vi "HFRR ADV v036 new software.vi"() -> ()   [LabVIEW 2025] (continued)
                        n2404 = local write "EVENT LOG"(w3467) -> ()
                      }
                      frame #22 {
                        n2405 = Wait (ms)(milliseconds to wait=u32 50) -> ()  [unwired: 1 out]
                      }
                      frame #23 {
                        n2406 = local read "NORMAL LOAD"() -> (w3471:dbl)
                        n2407 = Number To Fractional String(number=w3471, precision (6)=i16 2) -> (F-format string=w3472:string)  [unwired: 2 in]
                        n2408 = Concatenate Strings("Applied Load [grams] :" ("Content"), w3472) -> (w3474:string)
                        n2409 = local read "EVENT LOG"() -> (w3476:string)
                        n2410 = call "Event Log.vi"("Content"=w3474, "EVENT LOG"=w3476) -> ("EVENT LOG"=w3475:string)  [unwired: 8 in, 1 out]
                        n2411 = local write "EVENT LOG"(w3475) -> ()
                      }
                      frame #24 {
                        n2412 = Wait (ms)(milliseconds to wait=u32 50) -> ()  [unwired: 1 out]
                      }
                      frame #25 {
                        n2413 = local read "Set Strk"() -> (w3479:dbl)
                        n2414 = Number To Fractional String(number=w3479, precision (6)=i16 2) -> (F-format string=w3480:string)  [unwired: 2 in]
                        n2415 = Concatenate Strings("Set Stroke [mm] :" ("Content"), w3480) -> (w3482:string)
                        n2416 = local read "EVENT LOG"() -> (w3484:string)
                        n2417 = call "Event Log.vi"("Content"=w3482, "EVENT LOG"=w3484) -> ("EVENT LOG"=w3483:string)  [unwired: 8 in, 1 out]
                        n2418 = local write "EVENT LOG"(w3483) -> ()
                      }
                      frame #26 {
                        n2419 = Wait (ms)(milliseconds to wait=u32 50) -> ()  [unwired: 1 out]
                      }
                      frame #27 {
                        n2420 = local read "Set Temp"() -> (w3487:dbl)
                        n2421 = Number To Fractional String(number=w3487, precision (6)=i16 2) -> (F-format string=w3488:string)  [unwired: 2 in]
                        n2422 = Concatenate Strings("Set Temperature [deg C] :" ("Content"), w3488) -> (w3490:string)
                        n2423 = local read "EVENT LOG"() -> (w3492:string)
                        n2424 = call "Event Log.vi"("Content"=w3490, "EVENT LOG"=w3492) -> ("EVENT LOG"=w3491:string)  [unwired: 8 in, 1 out]
                        n2425 = local write "EVENT LOG"(w3491) -> ()
                      }
                      frame #28 {
                        n2426 = Wait (ms)(milliseconds to wait=u32 50) -> ()  [unwired: 1 out]
                      }
                      frame #29 {
                        n2427 = local read "Set Rh"() -> (w3495:dbl)
                        n2428 = Number To Fractional String(number=w3495, precision (6)=i16 2) -> (F-format string=w3496:string)  [unwired: 2 in]
                        n2429 = Concatenate Strings("Set Humidity [%RH] :" ("Content"), w3496) -> (w3498:string)
                        n2430 = local read "EVENT LOG"() -> (w3500:string)
                        n2431 = call "Event Log.vi"("Content"=w3498, "EVENT LOG"=w3500) -> ("EVENT LOG"=w3499:string)  [unwired: 8 in, 1 out]
                        n2432 = local write "EVENT LOG"(w3499) -> ()
                      }
                      frame #30 {
                        n2433 = Wait (ms)(milliseconds to wait=u32 50) -> ()  [unwired: 1 out]
                      }
                      frame #31 {
                        n2434 = local read "test time"() -> (w3503:dbl)
                        n2435 = Number To Fractional String(number=w3503, precision (6)=i16 1) -> (F-format string=w3504:string)  [unwired: 2 in]
                        n2436 = Concatenate Strings("Test Duration [mins] :" ("Content"), w3504) -> (w3506:string)
                        n2437 = local read "EVENT LOG"() -> (w3508:string)
                        n2438 = call "Event Log.vi"("Content"=w3506, "EVENT LOG"=w3508) -> ("EVENT LOG"=w3507:string)  [unwired: 8 in, 1 out]
                        n2439 = local write "EVENT LOG"(w3507) -> ()
                      }
                      frame #32 {
                        w3509 = dbl[] [] ("History Data")
                        w3510 = cluster{"y":dbl, dbl, "y":dbl}[] [] ("History Data")
                        w3511 = FALSE ("Visible")
                        n2440 = property on="Stroke ( mm )" class="WFChart (strict)"("History Data"=w3510) -> ()  [unwired: 2 in, 2 out]
                        n2441 = property on="Humidity ( %RH ) 2" class="WFChart (strict)"("History Data"=w3509) -> ()  [unwired: 2 in, 2 out]
                        n2442 = property on="Temperature ( Deg C )" class="WFChart (strict)"("History Data"=w3509) -> ()  [unwired: 2 in, 2 out]
                        n2443 = property on="Electrical Contact Resistance ( % )" class="WFChart (strict)"("History Data"=w3509) -> ()  [unwired: 2 in, 2 out]
                        n2444 = property on="Coefficient of Friction" class="WFChart (strict)"("History Data"=w3509) -> ()  [unwired: 2 in, 2 out]
                        n2445 = property on="Frictional Force ( N )" class="WFChart (strict)"("History Data"=w3509) -> ()  [unwired: 2 in, 2 out]
                        n2446 = property on="Coefficient of Friction" class="WFChart (strict)"("History Data"=w3509) -> ()  [unwired: 2 in, 2 out]
                        n2447 = property on="Frictional Force ( N )" class="WFChart (strict)"("History Data"=w3509) -> ()  [unwired: 2 in, 2 out]
                        n2448 = property on="Electrical Contact Resistance ( % )" class="WFChart (strict)"("History Data"=w3509) -> ()  [unwired: 2 in, 2 out]
                        n2449 = property on="Stroke ( mm )" class="WFChart (strict)"("History Data"=w3510) -> ()  [unwired: 2 in, 2 out]
                        n2450 = property on="Temperature ( Deg C )" class="WFChart (strict)"("History Data"=w3509) -> ()  [unwired: 2 in, 2 out]
                        n2451 = property on="Service Password Log" class="Str"("Visible"=w3511) -> ()  [unwired: 2 in, 2 out]
                        n2452 = property on="Password 3" class="Clust (strict)"("Visible"=w3511) -> ()  [unwired: 2 in, 2 out]
                      }
                    }
                    "TEST FILE NAM,E SAVED" <- TRUE ("TEST FILE NAM,E SAVED")
                  }
                }
              }
            }
          }
        }
        n2453 = local write "Test \nStatus"(w2890) -> ()
        n2454 = local write "Save"(w2890) -> ()
        n2455 = local read "Main Tab"() -> (w2884:T2)
        n2456 = case shown="True" w2887 {
          frame False {
            n2457 = local read "Rt 3"() -> (w2955:bool)
            n2458 = case shown="True" w2955 {
              frame False {
              }
              frame True {
                n2459 = local write "Rt 3"(FALSE ("Rt 3")) -> ()
              }
            }
            "Rt" <- TRUE ("Rt")
            "Rt 2" <- FALSE ("Rt")
          }
          frame True {
            n2460 = local read "Rt"() -> (w2961:bool)
            n2461 = local write "Rt 2"(TRUE ("Rt 2")) -> ()
            n2462 = case shown="True" w2961 {
              frame False {
              }
              frame True {
                n2463 = local write "Rt"(FALSE ("Rt")) -> ()
              }
            }
            "Rt 3" <- TRUE ("Rt 3")
          }
        }
        n2464 = case shown="\"Acquire\"" w2884 {
          tunnel: w2886 -> [_ w2990]
          frame Default {
            w2989 = 0.0 ("output")
            n2465 = local write "PID-out"(w2989) -> ()
            n2466 = local write "Frequency ( Hz )"(w2989) -> ()
            n2467 = local write "STROKE Initialize"(TRUE ("STROKE Initialize")) -> ()
          }
          frame "Acquire" {
            n2468 = stacked-sequence {
              frame #0 {
                n2469 = local read "Auto Start Test"() -> (w2992:bool)
                n2470 = case shown="True" w2992 {
                  tunnel: "RUN" -> [w3013 w3016]
                  tunnel: [w3013 w3015] -> w2993
                  frame False {
                  }
                  frame True {
                    n2471 = local read "Auto Start Temp"() -> (w3014:bool)
                    n2472 = Or(x=w3016, y=w3014) -> (x .or. y?=w3015:bool)
                  }
                }
                n2473 = local read "clk"() -> (w3012:dbl)
                n2474 = local read "Save"() -> (w3008:bool)
                n2475 = Equal?(x=w3012, y=0.0) -> (x = y?=w3009:bool)
                n2476 = And(x=w3009, y=w3008) -> (x .and. y?=w3010:bool)
                n2477 = Not(x="Engage") -> (.not. x?=w2999:bool)
                n2478 = case shown="False" w2993 {
                  tunnel: [0.0 w3039] -> w2995
                  frame False {
                    (unwired) TRUE ("Visible")
                    n2479 = local read "Auto Start Test"() -> (w3020:bool)
                    n2480 = local write "Start Time"(TRUE ("Start Time")) -> ()
                    n2481 = property on="Stroke 2" class="DigNum (strict)"("Visible"=FALSE) -> ()  [unwired: 2 in, 2 out]
                    n2482 = case shown="False" w3020 {
                      frame False {
                        n2483 = property on="Heater Button" class="Bool (strict)"("DisabledEnum"=T19."Enabled" ("Disabled")) -> ()  [unwired: 2 in, 2 out]
                        n2484 = property on="Humidity" class="Bool (strict)"("DisabledEnum"=T19."Enabled" ("Disabled")) -> ()  [unwired: 2 in, 2 out]
                      }
                      frame True {
                      }
                    }
                    n2485 = case shown="False" "TestCompFlg" {
                      frame False {
                        n2486 = local read "StartFlg"() -> (w3028:bool)
                        n2487 = case shown="True" w3028 {
                          frame False {
                          }
                          frame True {
                            n2488 = stacked-sequence {
                              frame #0 {
                                n2489 = local read "EVENT LOG"() -> (w3032:string)
                                n2490 = call "Event Log.vi"("Content"="Test was interrupted", "EVENT LOG"=w3032) -> ("EVENT LOG"=w3033:string)  [unwired: 8 in, 1 out]
                                n2491 = local write "EVENT LOG"(w3033) -> ()
                                n2492 = property on="RUN" class="Bool (strict)"("Visible"=TRUE) -> ()  [unwired: 2 in, 2 out]
                                n2493 = property on="Auto Start Test" class="Bool (strict)"("Visible"=TRUE) -> ()  [unwired: 2 in, 2 out]
                              }
                              frame #1 {
                                w3035 = FALSE ("StartFlg")
                                n2494 = property on="Heater Button" class="Bool (strict)"("Val(Sgnl)"=FALSE ("Value (Signaling)")) -> ()  [unwired: 2 in, 2 out]
                                n2495 = local write "Heater Button"(w3035) -> ()
                                n2496 = local write "StartFlg"(w3035) -> ()
                                n2497 = local write "Humidity"(w3035) -> ()
                              }
                              frame #2 {
                                n2498 = local write "Due Write"("VC;0" ("Command")) -> ()
                              }
                              frame #3 {
                                n2499 = Wait (ms)(milliseconds to wait=u32 1500) -> ()  [unwired: 1 out]
                              }
                              frame #4 {
                                n2500 = local write "Due Write"("HE;0" ("Command")) -> ()
                              }
                            }
                          }
                        }
                      }
                      frame True {
                      }
                    }
                    n2501 = local write "String 14"("Test will autostart once parameters reach the set value." ("String 14")) -> ()
                  }
                  frame True {
                    (unwired) FALSE ("Visible")
                    n2502 = property on="Stroke 2" class="DigNum (strict)"("Visible"=TRUE) -> ()  [unwired: 2 in, 2 out]
                    n2503 = property on="STOP 2" class="Bool (strict)"("Disabled"=u8 2) -> ()  [unwired: 2 in, 2 out]
                    n2504 = local write "String 14"(" Running....." ("String 14")) -> ()
                    n2505 = property on="Heater Button" class="Bool (strict)"("DisabledEnum"=T19."Disabled and Grayed Out" ("Disabled")) -> ()  [unwired: 2 in, 2 out]
                    n2506 = property on="Humidity" class="Bool (strict)"("DisabledEnum"=T19."Disabled and Grayed Out" ("Disabled")) -> ()  [unwired: 2 in, 2 out]
                    n2507 = case shown="True" "Start Time" {
                      selector: "Start Time" -> [_ w3058]
                      frame False {
                      }
                      frame True {
                        n2508 = Not(x=w3058) -> (.not. x?=w3057:bool)
                        n2509 = local write "Start Time"(w3057) -> ()
                        n2510 = local read "EVENT LOG"() -> (w3059:string)
                        n2511 = call "Event Log.vi"("Content"="Test in progress", "EVENT LOG"=w3059) -> ("EVENT LOG"=w3061:string)  [unwired: 8 in, 1 out]
                        n2512 = local write "EVENT LOG"(w3061) -> ()
                      }
                    }
                    n2513 = disable-structure shown="Enabled" {
                      disable-tunnel: [w3050 w3056] -> w3039
                      frame Disabled {
                        n2514 = local read "Set Hz"() -> (w3053:dbl)
                        n2515 = call <vilib>:"Uniform White Noise Waveform.vi"() -> ("signal out"=w3052:waveform(dbl))  [unwired: 10 in, 1 out]
                        n2516 = Random Number (0-1)() -> (number: 0 to 1=w3049:dbl)
                        n2517 = Add(x=w3053, y=w3052) -> (x+y=w3051:waveform(dbl))
                        n2518 = Multiply(x=ext 0.01 ("y"), y=w3049) -> (x*y=w3047:ext)
                        n2519 = Multiply(x=w3051, y=w3047) -> (x*y=w3050:waveform(ext))
                      }
                      frame Enabled {
                        n2520 = call-poly <vilib>:"Random Number (Range).vi"("lower bound (0)"=49.89, "upper bound (100)"=50.8) -> ("number"=w3056:dbl)  [unwired: 9 in]
                      }
                    }
                    "StartFlg" <- TRUE ("StartFlg")
                  }
                }
                n2521 = case shown="True" w3010 {
                  frame False {
                  }
                  frame True {
                    n2522 = local write "clk"(10.0 ("clk")) -> ()
                    n2523 = Get Date/Time In Seconds() -> (seconds since 1Jan1904=w3064:timestamp)
                    n2524 = To Double Precision Float(number=w3064) -> (double precision float=w3062:dbl)
                    n2525 = local write "acq timer"(w3062) -> ()
                    n2526 = local write "act save time"(w3062) -> ()
                  }
                }
                n2527 = call "Elapsed Time"("Time Target (s)"="Countdown", "Reset"=w2999) -> ("Elapsed Time (s)"=w3004:dbl, "Time has Elapsed"=w3002:bool)  [unwired: 10 in, 6 out]
                "Countdown 2" <- w3004
                n2528 = Subtract(x=w3004, y=2.0) -> (x-y=w3007:dbl)
                n2529 = Less?(x=w3007, y="Countdown") -> (x < y?=w3005:bool)
                n2530 = And(x=w3005, y=w3002) -> (x .and. y?=w3001:bool)
                n2531 = case shown="True" w3001 {
                  frame False {
                  }
                  frame True {
                    (unwired) dbl[] [] ("History Data")
                    n2532 = local write "Engage"(FALSE ("Engage")) -> ()
                    n2533 = local write "RUN"(TRUE ("RUN")) -> ()
                    n2534 = local read "Humidity ( %RH )"() -> (→"Rh Before":dbl)
                  }
                }
                n2535 = local read "Test \nStatus"() -> (w2997:bool)
                n2536 = Select(t=w2995, s=w2997, f=0.0) -> (s? t:f=w2996:dbl)
                n2537 = local write "Frequency ( Hz )"(w2996) -> ()
              }
              frame #1 {
                w3087 = 1000000.0 ("x")
                # "HC;1/0\nST;VALUE"
                # "Elapsed time\ncof\nstroke\nAir temp\nTemp\nHumidity"
                # "acq timer\n\nact save time"
                # "convert to microseconds"
                n2538 = local read "COUNT"() -> (w3070:i32)
                n2539 = local read "Rate"() -> (w3083:dbl)
                n2540 = Divide(x=w3087, y=w3083) -> (x/y=w3088:dbl)
                n2541 = Greater Or Equal?(x=w3070, y=250) -> (x >= y?=w3069:bool)
                n2542 = Get Date/Time In Seconds() -> (seconds since 1Jan1904=w3090:timestamp)
                n2543 = case shown="True" w3069 {
                  frame False {
                    n2544 = local read "COUNT"() -> (w3091:i32)
                    n2545 = Increment(x=w3091) -> (x+1=w3092:i32)
                    n2546 = local write "COUNT"(w3092) -> ()
                  }
                  frame True {
                    n2547 = local write "COUNT"(0 ("COUNT")) -> ()
                  }
                }
                n2548 = local read "Samplingtime 2"() -> (w3068:dbl)
                n2549 = local read "act save time"() -> (w3085:dbl)
                n2550 = Divide(x=w3088, y=w3087) -> (x/y=w3086:dbl)
                n2551 = To Double Precision Float(number=w3090) -> (double precision float=w3079:dbl)
                n2552 = Add(x=w3085, y=w3068) -> (x+y=w3084:dbl)
                n2553 = local read "acq timer"() -> (w3089:dbl)
                n2554 = local read "COUNT"() -> (w3072:i32)
                n2555 = Greater Or Equal?(x=w3079, y=w3084) -> (x >= y?=w3067:bool)
                n2556 = Multiply(x=w3086, y=w3072) -> (x*y=w3078:dbl)
                n2557 = Subtract(x=w3079, y=w3089) -> (x-y=w3081:dbl)
                n2558 = local read "Save"() -> (w3082:bool)
                n2559 = Add(x=w3081, y=w3078) -> (x+y=w3065:dbl)
                "Elapsed time 3" <- w3065
                n2560 = And(x=w3067, y=w3082) -> (x .and. y?=w3080:bool)
                n2561 = Divide(x=w3065, y=60.0) -> (x/y=w3076:dbl)
                n2562 = local read "Test \nStatus"() -> (w3066:bool)
                n2563 = local read "clk"() -> (w3073:dbl)
                n2564 = Equal?(x=w3073, y=10.0) -> (x = y?=w3075:bool)
                n2565 = case shown="True" w3080 {
                  tunnel: w3079 -> [_ w3211]
                  tunnel: [FALSE ("Boolean 2") TRUE ("Boolean 2")] -> _
                  frame False {
                  }
                  frame True {
                    w3165 = ";" ("Substring")
                    # "Pid out/\nFreq response value"
                    n2566 = local write "act save time"(w3211) -> ()
                    n2567 = local read "FILE"() -> (w3159:string)
                    n2568 = call "file check.vi"("file name in"=w3159) -> ("error out"=w3162:errorcluster, "file name out"=w3157:string)  [unwired: 9 in]
                    n2569 = local read "LVDT STROKE"() -> (w3154:dbl)
                    n2570 = local read "Add up Stroke"() -> (w3152:dbl)
                    n2571 = call "FILE PATH CREATION.vi"("error in"=w3162, "FILE NAME :"=w3157) -> ("FILE OUT"=w3160:path)  [unwired: 8 in, 1 out]
                    n2572 = local read "STROKE Initialize"() -> (w3147:bool)
                    n2573 = Concatenate Strings(w3157, ".dgf" ("Substring")) -> (w3161:string)
                    n2574 = Subtract(x=w3154, y=w3152) -> (x-y=w3153:dbl)
                    n2575 = Absolute Value(x=w3153) -> (abs(x)=w3150:dbl)
                    n2576 = local read "FF 2"() -> (→"Frictional Force ( N )" →"Frictional Force ( N )":dbl)
                    n2577 = Build Path(base path=w3160, name or relative path=w3161) -> (appended path=w3156:path)
                    n2578 = flat-sequence {
                      tunnel: w3150 -> [w3216]
                      tunnel: [w3215] -> w3148
                      tunnel: w3147 -> [w3213]
                      tunnel: [w3218] -> w3149
                      tunnel: w3148 -> [w3218]
                      frame #0 {
                        n2579 = call <vilib>:"Mean PtByPt.vi"("x"=w3216, "sample length"="STROKE FILTER", "initialize"=w3213) -> ("mean"=w3215:dbl)  [unwired: 1 in, 1 out]
                      }
                      frame #1 {
                        "STROKE Initialize" <- FALSE ("STROKE Initialize")
                      }
                    }
                    n2580 = local read "COF 2"() -> (w3170:dbl)
                    "Coefficient of Friction" <- w3170
                    "COF 4" <- w3170
                    "Coefficient of Friction" <- w3170
                    n2581 = local read "TEMP"() -> (w3173:dbl)
                    "Temperature ( Deg C )" <- w3173
                    n2582 = local read "Humidity ( %RH )"() -> (w3172:dbl)
                    "Humidity ( %RH ) 2" <- w3172
                    n2583 = local read "Frequency ( Hz )"() -> (w3179:dbl)
                    n2584 = local read "LVDT STROKE DISPLAY"() -> (w3151:dbl)
                    n2585 = local read "Elapsed time"() -> (w3204:dbl)
                    n2586 = local read "AIR TEMP"() -> (w3177:dbl)
                    n2587 = local read "PID-out"() -> (w3182:dbl)
                    n2588 = local write "Temperature ( Deg C )"(w3173) -> ()
                    n2589 = Number To Fractional String(number=w3151, width (-)=i16 9 ("precision (6)"), precision (6)=i16 6) -> (F-format string=w3197:string)  [unwired: 1 in]
                    n2590 = Number To Fractional String(number=w3177, width (-)=i16 9 ("precision (6)"), precision (6)=i16 3) -> (F-format string=w3196:string)  [unwired: 1 in]
                    n2591 = Number To Fractional String(number=w3173, width (-)=i16 9 ("precision (6)"), precision (6)=i16 3) -> (F-format string=w3193:string)  [unwired: 1 in]
                    n2592 = Number To Fractional String(number=w3172, width (-)=i16 9 ("precision (6)"), precision (6)=i16 3) -> (F-format string=w3190:string)  [unwired: 1 in]
                    n2593 = Number To Fractional String(number=0.0, width (-)=i16 9 ("precision (6)"), precision (6)=i16 3) -> (F-format string=w3187:string)  [unwired: 1 in]
                    n2594 = Number To Fractional String(number=w3182, width (-)=i16 9 ("precision (6)"), precision (6)=i16 3) -> (F-format string=w3183:string)  [unwired: 1 in]
                    n2595 = Number To Fractional String(number=w3179, width (-)=i16 9 ("precision (6)"), precision (6)=i16 3) -> (F-format string=w3178:string)  [unwired: 1 in]
                    n2596 = Number To Fractional String(number=w3170, width (-)=i16 9 ("precision (6)"), precision (6)=i16 6) -> (F-format string=w3205:string)  [unwired: 1 in]
                    n2597 = Number To Fractional String(number=w3204, width (-)=i16 14 ("precision (6)"), precision (6)=i16 3) -> (F-format string=w3206:string)  [unwired: 1 in]
                    n2598 = Bundle("y"=1.02, "LVDT STROKE DISPLAY"=w3151, "y"=0.98) -> (w3171:T30)  [unwired: 1 in]
                    n2599 = Number To Fractional String(number="Ambient Humidity :", width (-)=i16 9 ("precision (6)"), precision (6)=i16 6) -> (F-format string=w3163:string)  [unwired: 1 in]
                    n2600 = local read "RUN"() -> (w3169:bool)
                    n2601 = case shown="True" w3169 {
                      tunnel: w3171 -> [_ w3222]
                      tunnel: w3151 -> [_ w3221]
                      tunnel: w3151 -> [_ w3219]
                      tunnel: w3151 -> [_ w3220]
                      frame False {
                      }
                      frame True {
                        "Stroke ( mm )" <- w3222
                        "Stroke ( mm )" <- w3222
                        "Stroke 4" <- w3221
                        "Stroke 3" <- w3219
                        "Stroke 2" <- w3220
                        "measured_stroke" <- w3219
                      }
                    }
                    n2602 = Concatenate Strings(w3206, w3165, w3205, w3165, w3197, w3165, w3196, w3165, w3193, w3165, w3190, w3165, w3187, w3165, w3183, w3165, w3178, w3165, w3163, "\r") -> (w3203:string)
                    n2603 = call <vilib>:"Write Characters To File.vi"("append to file? (new file:F)"=TRUE, "character string"=w3203, "file path (dialog if empty)"=w3156) -> ()  [unwired: 2 in, 1 out]
                    "refresh flag" <- TRUE ("refresh flag")
                    "LVDT STROKE Actual" <- w3149
                  }
                }
                n2604 = case shown="True" w3066 {
                  tunnel: w3076 -> [_ w3102]
                  tunnel: w3081 -> [_ w3112]
                  tunnel: [0.0 w3108] -> _
                  tunnel: w3075 -> [_ w3107]
                  tunnel: [0.0 w3106] -> _
                  tunnel: w3065 -> [_ w3106]
                  tunnel: w3079 -> [w3095 _]
                  frame False {
                    n2605 = local write "acq timer"(w3095) -> ()
                    n2606 = local write "Test Duration Status"(0.0 ("Test Duration Status")) -> ()
                  }
                  frame True {
                    n2607 = local read "Set Hz"() -> (w3109:dbl)
                    n2608 = local write "Elapsed time"(w3102) -> ()
                    n2609 = local read "test time"() -> (w3101:dbl)
                    n2610 = Multiply(x=w3112, y=w3109) -> (x*y=w3111:dbl)
                    n2611 = case shown="False" w3107 {
                      tunnel: w3111 -> [w3113 _]
                      tunnel: [w3113 1.0] -> w3108
                      frame False {
                        n2612 = local write "Cycles elapsed"(w3113) -> ()
                      }
                      frame True {
                      }
                    }
                    n2613 = Greater?(x=w3102, y=w3101) -> (0:w3110:bool)
                    n2614 = Subtract(x=w3101, y=w3102) -> (x-y=w3100:dbl)
                    n2615 = Multiply(x=w3100, y=60.0) -> (x*y=w3099:dbl)
                    n2616 = local write "Time Remaining"(w3099) -> ()
                    n2617 = local write "Remaining Time"(w3099) -> ()
                    n2618 = case shown="True" w3110 {
                      frame False {
                      }
                      frame True {
                        n2619 = stacked-sequence {
                          frame #0 {
                            w3118 = T19."Enabled" ("Disabled")
                            w3117 = FALSE ("TEST FILE NAM,E SAVED")
                            w3119 = "" ("FILE")
                            w3120 = TRUE ("Visible")
                            n2620 = local write "Humidity"(FALSE ("Humidity")) -> ()
                            n2621 = local write "RUN"(FALSE ("OK Button 2")) -> ()
                            n2622 = local write "Heater Button"(FALSE ("Heater Button")) -> ()
                            n2623 = local write "Auto Start Test"(FALSE ("Auto Start Test")) -> ()
                            n2624 = local write "TestCompFlg"(TRUE ("StpFlg")) -> ()
                            n2625 = local read "Humidity ( %RH )"() -> (→"Rh After":dbl)
                            n2626 = property on="STOP 2" class="Bool (strict)"("Disabled"=u8 0) -> ()  [unwired: 2 in, 2 out]
                            n2627 = local read "EVENT LOG"() -> (w3125:string)
                            n2628 = call "Event Log.vi"("Content"="Test Completed", "EVENT LOG"=w3125) -> ("EVENT LOG"=w3124:string)  [unwired: 8 in, 1 out]
                            n2629 = property on="RUN" class="Bool (strict)"("Visible"=w3120) -> ()  [unwired: 2 in, 2 out]
                            n2630 = property on="Auto Start Test" class="Bool (strict)"("Visible"=w3120) -> ()  [unwired: 2 in, 2 out]
                            n2631 = local write "Batch Ref Num :"(w3119) -> ()
                            n2632 = local write "FILE"(w3119) -> ()
                            n2633 = local write "EVENT LOG"(w3124) -> ()
                            n2634 = local write "TEST FILE NAM,E SAVED"(w3117) -> ()
                            n2635 = local write "Fuel Discription :"(w3119) -> ()
                            n2636 = local write "START TEMP"(w3117) -> ()
                            n2637 = local write "Remarks :"(w3119) -> ()
                            n2638 = local write "Main Dashboard Buttons"(T1."Imaging" ("Main Dashboard Buttons")) -> ()
                            n2639 = local write "Main Tab"(T2."Adv Scar" ("Main Tab")) -> ()
                            n2640 = property on="FRICVALZ 2" class="Bool (strict)"("DisabledEnum"=w3118) -> ()  [unwired: 2 in, 2 out]
                            n2641 = property on="FRICVALZ 3" class="Bool (strict)"("DisabledEnum"=w3118) -> ()  [unwired: 2 in, 2 out]
                            n2642 = property on="FRICVALZ 4" class="Bool (strict)"("DisabledEnum"=w3118) -> ()  [unwired: 2 in, 2 out]
                          }
                          frame #1 {
                            n2643 = Wait (ms)(milliseconds to wait=u32 1500) -> ()  [unwired: 1 out]
                          }
                          frame #2 {
                            n2644 = local read "WriteHumidity"() -> (w3134:string[])
                            n2645 = Insert Into Array(array=w3134, new element="R;1" ("new element/subarray")) -> (w3132:string[])  [unwired: 1 in]
                            n2646 = local write "Due Write"("VC;0") -> ()
                            n2647 = local write "WriteHumidity"(w3132) -> ()
                          }
                          frame #3 {
                            n2648 = Wait (ms)(milliseconds to wait=u32 1500) -> ()  [unwired: 1 out]
                          }
                          frame #4 {
                            n2649 = local read "WriteHumidity"() -> (w3139:string[])
                            n2650 = Insert Into Array(array=w3139, new element="R;1" ("new element/subarray")) -> (w3138:string[])  [unwired: 1 in]
                            n2651 = local write "Due Write"("VC;0") -> ()
                            n2652 = local write "WriteHumidity"(w3138) -> ()
                          }
                          frame #5 {
                            n2653 = Wait (ms)(milliseconds to wait=u32 1500) -> ()  [unwired: 1 out]
                          }
                          frame #6 {
                            n2654 = local write "Due Write"("ST;0") -> ()
                          }
                          frame #7 {
                            n2655 = local write "measured_stroke"(0.0 ("measured_stroke")) -> ()
                            n2656 = Wait (ms)(milliseconds to wait=u32 1500) -> ()  [unwired: 1 out]
                          }
                          frame #8 {
                            n2657 = local write "Due Write"("HE;0") -> ()
                          }
                        }
                      }
                    }
                    n2658 = Divide(x=w3102, y=w3101) -> (x/y=w3105:dbl)
                    n2659 = Multiply(x=w3105, y=100.0) -> (x*y=w3103:dbl)
                    n2660 = local write "Test Duration Status"(w3103) -> ()
                  }
                }
              }
              frame #2 {
                n2661 = case shown="True" "Heater Button" {
                  tunnel: [0.0 ("output") w3245] -> w3223
                  frame False {
                    w3226 = TRUE ("tmpchk")
                    n2662 = local read "TEMP"() -> (w3227:dbl)
                    n2663 = local write "Temp ini"(w3227) -> ()
                    n2664 = local write "Reset 4"(w3226) -> ()
                    n2665 = local write "tmpchk"(w3226) -> ()
                    n2666 = local write "reinit"(TRUE ("reinit")) -> ()
                    n2667 = local write "manual temp log"(TRUE ("manual temp log")) -> ()
                  }
                  frame True {
                    # "Logic to turn off\nthe heater when \ntemp is not rising.\nTime - 60 sec\nDelta t- 5°c"
                    n2668 = local read "Temp ini"() -> (w3234:dbl)
                    n2669 = local read "Auto Start Test"() -> (w3230:bool)
                    n2670 = Less?(x=w3234, y=53.0) -> (x < y?=w3232:bool)
                    n2671 = case shown="False" w3230 {
                      frame False {
                        n2672 = local read "Set Temp"() -> (w3254:dbl)
                        n2673 = local read "TEMP"() -> (w3253:dbl)
                        n2674 = Subtract(x=w3254, y=w3253) -> (x-y=w3252:dbl)
                        n2675 = Absolute Value(x=w3252) -> (abs(x)=w3251:dbl)
                        n2676 = Less?(x=w3251, y=0.5) -> (x < y?=w3249:bool)
                        n2677 = case shown="True" w3249 {
                          tunnel: "manual temp log" -> [_ w3255]
                          frame False {
                          }
                          frame True {
                            n2678 = case shown="True" w3255 {
                              selector: w3255 -> [_ w3256]
                              frame False {
                              }
                              frame True {
                                # "#Event log"
                                n2679 = Not(x=w3256) -> (.not. x?=w3257:bool)
                                n2680 = local write "manual temp log"(w3257) -> ()
                                n2681 = local read "EVENT LOG"() -> (w3260:string)
                                n2682 = call "Event Log.vi"("Content"="Target Temperature reached", "EVENT LOG"=w3260) -> ("EVENT LOG"=w3259:string)  [unwired: 8 in, 1 out]
                                n2683 = local write "EVENT LOG"(w3259) -> ()
                              }
                            }
                          }
                        }
                      }
                      frame True {
                        n2684 = local write "manual temp log"(TRUE ("manual temp log")) -> ()
                      }
                    }
                    n2685 = And(x="tmpchk", y=w3232) -> (x .and. y?=w3235:bool)
                    n2686 = case shown="True" w3235 {
                      frame False {
                      }
                      frame True {
                        n2687 = call "Elapsed Time8"("Time Target (s)"=300.0, "Reset"="Reset 4") -> ("Time has Elapsed"=w3262:bool)  [unwired: 10 in, 7 out]
                        n2688 = flat-sequence {
                          tunnel: w3262 -> [_]
                          frame #0 {
                            n2689 = local write "Reset 4"(FALSE ("Reset 4")) -> ()
                          }
                        }
                        n2690 = case shown="True" w3262 {
                          frame False {
                          }
                          frame True {
                            n2691 = local read "Temp ini"() -> (w3269:dbl)
                            n2692 = Add(x=w3269, y=5.0) -> (x+y=w3267:dbl)
                            n2693 = local read "TEMP"() -> (w3270:dbl)
                            n2694 = Greater?(x=w3270, y=w3267) -> (0:w3268:bool)
                            n2695 = case shown="False" w3268 {
                              frame False {
                                n2696 = local write "Heater Button"(FALSE ("Heater Button")) -> ()
                              }
                              frame True {
                                n2697 = local write "tmpchk"(FALSE ("tmpchk")) -> ()
                              }
                            }
                          }
                        }
                      }
                    }
                    n2698 = local read "Set Temp"() -> (w3243:dbl)
                    n2699 = local read "TEMP"() -> (w3237:dbl)
                    n2700 = call-poly <vilib>:"PID.vi"("reinitialize? (F)"="reinit", "dt (s)"=-1.0, "process variable"=w3237, "setpoint"=w3243) -> ("output"=w3240:dbl)  [unwired: 6 in, 1 out]
                    n2701 = Subtract(x=w3243, y=w3237) -> (x-y=w3244:dbl)
                    n2702 = Add(x=w3243, y=0.5) -> (x+y=w3241:dbl)
                    n2703 = Greater Or Equal?(x=w3237, y=w3241) -> ()  [unwired: 1 out]
                    n2704 = Select(t=0.0, s=FALSE, f=w3240) -> (s? t:f=w3239:dbl)
                    "PID output" <- w3239
                    n2705 = flat-sequence {
                      tunnel: w3239 -> [w3273]
                      tunnel: [w3273] -> w3245
                      frame #0 {
                        n2706 = local write "reinit"(FALSE ("reinit")) -> ()
                      }
                    }
                    n2707 = Bundle(w3244, "output"=w3239, "TEMP"=w3237) -> ()  [unwired: 1 in, 1 out]
                  }
                }
                "PID-out" <- w3223
              }
              frame #3 {
                n2708 = local read "TEMP"() -> (w3275:dbl)
                n2709 = Greater Or Equal?(x=w3275, y="Set Temp 2") -> (x >= y?=w3280:bool)
                n2710 = case shown="True" w3280 {
                  tunnel: [FALSE TRUE] -> w3278
                  frame False {
                  }
                  frame True {
                  }
                }
                "Status 13" <- w3278
                n2711 = And(x=w3278, y="trip1 8") -> (x .and. y?=w3277:bool)
                n2712 = case shown="True" w3277 {
                  frame False {
                    n2713 = local write "Heater Trip Temp"(TRUE ("Heater Trip Temp")) -> ()
                  }
                  frame True {
                    w3283 = FALSE ("OK Button 2")
                    n2714 = case shown="True" "Heater Trip Temp" {
                      selector: "Heater Trip Temp" -> [_ w3285]
                      frame False {
                      }
                      frame True {
                        n2715 = Not(x=w3285) -> (.not. x?=w3284:bool)
                        n2716 = local read "EVENT LOG"() -> (w3288:string)
                        n2717 = local write "Heater Trip Temp"(w3284) -> ()
                        n2718 = call "Event Log.vi"("Content"="Heater Trip", "EVENT LOG"=w3288) -> ("EVENT LOG"=w3287:string)  [unwired: 8 in, 1 out]
                        n2719 = local write "EVENT LOG"(w3287) -> ()
                      }
                    }
                    n2720 = local write "RUN"(w3283) -> ()
                    n2721 = property on="Auto Start Test" class="Bool (strict)"("Value"=w3283) -> ()  [unwired: 2 in, 2 out]
                    n2722 = local write "Heater Button"(w3283) -> ()
                  }
                }
              }
            }
            n2723 = case shown="False" w2990 {
              frame False {
                n2724 = disable-structure shown="Disabled" {
                  frame Disabled {
                    n2725 = stacked-sequence {
                      frame #0 {
                        n2726 = local write "RUN"(FALSE ("OK Button 2")) -> ()
                      }
                      frame #1 {
                      }
                    }
                  }
                  frame Enabled {
                  }
                }
              }
              frame True {
              }
            }
          }
        }
        n2727 = local read "Reset Graph"() -> (w2883:bool)
        n2728 = case shown="True" w2883 {
          selector: w2883 -> [_ w2900]
          frame False {
          }
          frame True {
            w2914 = 0.0 ("X Scale.Range:Maximum")
            n2729 = Not(x=w2900) -> (.not. x?=w2899:bool)
            n2730 = local write "Reset Graph"(w2899) -> ()
            n2731 = property on="Electrical Contact Resistance ( % )" class="WFChart (strict)"("XScale.Maximum"=600.0 ("X Scale.Range:Maximum"), "XScale.Minimum"=0.0 ("X Scale.Range:Minimum"), "YScale.Maximum"=100.0 ("Y Scale.Range:Maximum"), "YScale.Minimum"=0.0 ("Y Scale.Range:Minimum")) -> ()  [unwired: 2 in, 2 out]
            n2732 = property on="Frictional Force ( N )" class="WFChart (strict)"("XScale.Maximum"=600.0 ("X Scale.Range:Maximum"), "XScale.Minimum"=0.0 ("X Scale.Range:Minimum"), "YScale.Maximum"=100.0 ("Y Scale.Range:Maximum"), "YScale.Minimum"=0.0 ("Y Scale.Range:Minimum")) -> ()  [unwired: 2 in, 2 out]
            n2733 = property on="Temperature ( Deg C )" class="WFChart (strict)"("XScale.Maximum"=600.0 ("X Scale.Range:Maximum"), "XScale.Minimum"=0.0 ("X Scale.Range:Minimum"), "YScale.Maximum"=100.0 ("Y Scale.Range:Maximum"), "YScale.Minimum"=0.0 ("Y Scale.Range:Minimum")) -> ()  [unwired: 2 in, 2 out]
            n2734 = property on="Stroke ( mm )" class="WFChart (strict)"("XScale.Maximum"=600.0 ("X Scale.Range:Maximum"), "XScale.Minimum"=0.0 ("X Scale.Range:Minimum"), "YScale.Maximum"=100.0 ("Y Scale.Range:Maximum"), "YScale.Minimum"=0.0 ("Y Scale.Range:Minimum")) -> ()  [unwired: 2 in, 2 out]
            n2735 = property on="Coefficient of Friction" class="WFChart (strict)"("XScale.Maximum"=600.0 ("X Scale.Range:Maximum"), "XScale.Minimum"=0.0 ("X Scale.Range:Minimum"), "YScale.Maximum"=100.0 ("Y Scale.Range:Maximum"), "YScale.Minimum"=0.0 ("Y Scale.Range:Minimum")) -> ()  [unwired: 2 in, 2 out]
            n2736 = property on="Electrical Contact Resistance ( % )" class="WFChart (strict)"("XScale.Minimum"=0.0 ("X Scale.Range:Minimum"), "XScale.Maximum"=600.0 ("X Scale.Range:Maximum"), "YScale.Minimum"=0.0 ("Y Scale.Range:Minimum"), "YScale.Maximum"=100.0 ("Y Scale.Range:Maximum")) -> ()  [unwired: 2 in, 2 out]
            n2737 = property on="Temperature ( Deg C )" class="WFChart (strict)"("XScale.Minimum"=0.0 ("X Scale.Range:Minimum"), "XScale.Maximum"=600.0 ("X Scale.Range:Maximum"), "YScale.Minimum"=0.0 ("Y Scale.Range:Minimum"), "YScale.Maximum"=100.0 ("Y Scale.Range:Maximum")) -> ()  [unwired: 2 in, 2 out]
            n2738 = property on="Coefficient of Friction" class="WFChart (strict)"("XScale.Minimum"=0.0 ("X Scale.Range:Minimum"), "XScale.Maximum"=600.0 ("X Scale.Range:Maximum"), "YScale.Maximum"=1.0 ("X Scale.Range:Minimum"), "YScale.Minimum"=0.0 ("X Scale.Range:Minimum")) -> ()  [unwired: 2 in, 2 out]
            n2739 = property on="Frictional Force ( N )" class="WFChart (strict)"("XScale.Maximum"=600.0 ("X Scale.Range:Maximum"), "XScale.Minimum"=w2914, "YScale.Maximum"=10.0 ("Y Scale.Range:Maximum"), "YScale.Minimum"=w2914) -> ()  [unwired: 2 in, 2 out]
            n2740 = property on="Stroke ( mm )" class="WFChart (strict)"("XScale.Maximum"=600.0 ("X Scale.Range:Maximum"), "XScale.Minimum"=0.0 ("X Scale.Range:Minimum"), "YScale.Maximum"=100.0 ("Y Scale.Range:Maximum"), "YScale.Minimum"=0.0 ("Y Scale.Range:Minimum")) -> ()  [unwired: 2 in, 2 out]
            n2741 = property on="Humidity ( %RH ) 2" class="WFChart (strict)"("XScale.Maximum"=600.0 ("X Scale.Range:Maximum"), "XScale.Minimum"=0.0 ("X Scale.Range:Minimum"), "YScale.Maximum"=100.0 ("Y Scale.Range:Maximum"), "YScale.Minimum"=0.0 ("Y Scale.Range:Minimum")) -> ()  [unwired: 2 in, 2 out]
          }
        }
      }
      frame "Compare Files" {
        # "Elapsed time\ncof\nstroke\nAir temp\nTemp\nHumidity"
        n2742 = case shown="True" "RSTV1 2" {
          frame False {
          }
          frame True {
            n2743 = property on="Humidity ( %RH )" class="XYGraph (strict)"("Y Scale.Display Format:Precision"=u8 0 ("Y Scale.Format & Precision:Precision")) -> ()  [unwired: 2 in, 2 out]
            n2744 = property on="Humidity ( %RH )" class="XYGraph (strict)"("X Scale.Range:Minimum"=0.0, "X Scale.Range:Maximum"=75.0, "Y Scale.Range:Minimum"=48.0, "Y Scale.Range:Maximum"=58.0) -> ()  [unwired: 2 in, 2 out]
          }
        }
        n2745 = case shown="True" "RST CP 2" {
          frame False {
          }
          frame True {
            n2746 = property on="XY Graph 13" class="XYGraph (strict)"("Y Scale.Display Format:Precision"=u8 0 ("Y Scale.Format & Precision:Precision")) -> ()  [unwired: 2 in, 2 out]
            n2747 = property on="XY Graph 13" class="XYGraph (strict)"("X Scale.Range:Minimum"=0.0, "X Scale.Range:Maximum"=75.0, "Y Scale.Range:Minimum"=0.0, "Y Scale.Range:Maximum"=100.0) -> ()  [unwired: 2 in, 2 out]
          }
        }
        n2748 = case shown="True" "RST CP" {
          frame False {
          }
          frame True {
            n2749 = property on="Sample Temperature ( °C )" class="XYGraph (strict)"("Y Scale.Display Format:Precision"=u8 2 ("Y Scale.Format & Precision:Precision")) -> ()  [unwired: 2 in, 2 out]
            n2750 = property on="Sample Temperature ( °C )" class="XYGraph (strict)"("X Scale.Range:Minimum"=0.0, "X Scale.Range:Maximum"=75.0, "Y Scale.Range:Minimum"=58.0, "Y Scale.Range:Maximum"=62.0) -> ()  [unwired: 2 in, 2 out]
          }
        }
        n2751 = case shown="True" "RSTV1 3" {
          frame False {
          }
          frame True {
            n2752 = property on="Air Temperature  ( °C )" class="XYGraph (strict)"("Y Scale.Display Format:Precision"=u8 2 ("Y Scale.Format & Precision:Precision")) -> ()  [unwired: 2 in, 2 out]
            n2753 = property on="Air Temperature  ( °C )" class="XYGraph (strict)"("X Scale.Range:Minimum"=0.0 ("Y Scale.Range:Minimum"), "X Scale.Range:Maximum"=75.0 ("Y Scale.Range:Maximum"), "Y Scale.Range:Minimum"=20.0 ("X Scale.Range:Minimum"), "Y Scale.Range:Maximum"=26.0 ("X Scale.Range:Maximum")) -> ()  [unwired: 2 in, 2 out]
          }
        }
        n2754 = case shown="True" "RSTV1 4" {
          frame False {
          }
          frame True {
            n2755 = property on="Stroke ( mm )" class="XYGraph (strict)"("Y Scale.Display Format:Precision"=u8 2 ("Y Scale.Format & Precision:Precision")) -> ()  [unwired: 2 in, 2 out]
            n2756 = property on="Stroke ( mm )" class="XYGraph (strict)"("X Scale.Range:Minimum"=0.0 ("Y Scale.Range:Maximum"), "X Scale.Range:Maximum"=75.0 ("X Scale.Range:Minimum"), "Y Scale.Range:Minimum"=0.98, "Y Scale.Range:Maximum"=1.02) -> ()  [unwired: 2 in, 2 out]
          }
        }
        n2757 = case shown="True" "rstv2" {
          frame False {
          }
          frame True {
            n2758 = property on="Coefficient Of Friction" class="XYGraph (strict)"("Y Scale.Display Format:Precision"=u8 3 ("Y Scale.Format & Precision:Precision")) -> ()  [unwired: 2 in, 2 out]
            n2759 = property on="Coefficient Of Friction" class="XYGraph (strict)"("X Scale.Range:Minimum"=0.0 ("Y Scale.Range:Maximum"), "X Scale.Range:Maximum"=75.0, "Y Scale.Range:Minimum"=0.0, "Y Scale.Range:Maximum"=1.0 ("X Scale.Range:Minimum")) -> ()  [unwired: 2 in, 2 out]
          }
        }
        n2760 = case shown="True" "RST CP 3" {
          frame False {
          }
          frame True {
            n2761 = property on="Air Temp ( °C ) vs Humidity ( % RH )" class="XYGraph (strict)"("X Scale.Range:Minimum"=18.0, "X Scale.Range:Maximum"=28.0 ("X Scale.Range:Minimum"), "Y Scale.Range:Minimum"=30.0 ("X Scale.Range:Minimum"), "Y Scale.Range:Maximum"=70.0 ("X Scale.Range:Minimum")) -> ()  [unwired: 2 in, 2 out]
          }
        }
        n2762 = case shown="True" "OPEN 1" {
          frame False {
          }
          frame True {
            (unwired) 0  # existing file
            w3564 = "Choose a datalog file to open"  # prompt
            n2763 = local write "OPEN 1"(FALSE ("OPEN 1")) -> ()
            n2764 = String To Path(string="C:\\LAB-IQ\\Data\\") -> (path=w3549:path)
            n2765 = File Dialog(6:"*.dgf" ("pattern"), 7:w3564, 11:w3549) -> (0:w3547:errorcluster, 3:w3555:path)  [unwired: 4 in, 2 out]
            n2766 = Unbundle(w3547) -> ()  [unwired: 3 out]
            n2767 = Strip Path(path=w3555) -> (name=w3554:string)  [unwired: 1 out]
            n2768 = Path To String(path=w3555) -> (string=w3550:string)
            "string1" <- w3550
            n2769 = Match Pattern(string=w3554, regular expression=".dgf") -> (before substring=→"String Control":string)  [unwired: 1 in, 3 out]
            n2770 = Match Pattern(string=w3550, regular expression=".dgf" ("substring (\"\")")) -> (before substring=w3560:string)  [unwired: 1 in, 3 out]
            n2771 = Concatenate Strings(w3560, ".duf" ("Substring")) -> (w3556:string)
            n2772 = String To Path(string=w3556) -> (path=w3561:path)
            n2773 = call <vilib>:"Read Characters From File.vi"("file path (dialog if empty)"=w3561, "start of read offset (chars.:0)"=60 ("start of read offset (chars.: 0)")) -> ("character string"=→"String Control 2":string)  [unwired: 4 in, 3 out]
          }
        }
        n2774 = case shown="True" "OPEN 2" {
          frame False {
          }
          frame True {
            (unwired) 0  # existing file
            w3582 = "Choose a datalog file to open"  # prompt
            n2775 = local write "OPEN 2"(FALSE ("OPEN 1")) -> ()
            n2776 = String To Path(string="C:\\LAB-IQ\\Data\\") -> (path=w3567:path)
            n2777 = File Dialog(6:"*.dgf" ("pattern"), 7:w3582, 11:w3567) -> (0:w3565:errorcluster, 3:w3573:path)  [unwired: 4 in, 2 out]
            n2778 = Unbundle(w3565) -> ()  [unwired: 3 out]
            n2779 = Strip Path(path=w3573) -> (name=w3571:string)  [unwired: 1 out]
            n2780 = Path To String(path=w3573) -> (string=w3568:string)
            "string1 2" <- w3568
            n2781 = Match Pattern(string=w3571, regular expression=".dgf") -> (before substring=→"String Control 3":string)  [unwired: 1 in, 3 out]
            n2782 = Match Pattern(string=w3568, regular expression=".dgf" ("substring (\"\")")) -> (before substring=w3579:string)  [unwired: 1 in, 3 out]
            n2783 = Concatenate Strings(w3579, ".duf" ("Substring")) -> (w3576:string)
            n2784 = String To Path(string=w3576) -> (path=w3574:path)
            n2785 = call <vilib>:"Read Characters From File.vi"("file path (dialog if empty)"=w3574, "start of read offset (chars.:0)"=60 ("start of read offset (chars.: 0)")) -> ("character string"=→"String Control 4":string)  [unwired: 4 in, 3 out]
          }
        }
        n2786 = case shown="True" "OPEN 3" {
          frame False {
          }
          frame True {
            (unwired) 0  # existing file
            w3600 = "Choose a datalog file to open"  # prompt
            n2787 = local write "OPEN 3"(FALSE ("OPEN 1")) -> ()
            n2788 = String To Path(string="C:\\LAB-IQ\\Data\\") -> (path=w3585:path)
            n2789 = File Dialog(6:"*.dgf" ("pattern"), 7:w3600, 11:w3585) -> (0:w3583:errorcluster, 3:w3591:path)  [unwired: 4 in, 2 out]
            n2790 = Unbundle(w3583) -> ()  [unwired: 3 out]
            n2791 = Strip Path(path=w3591) -> (name=w3589:string)  [unwired: 1 out]
            n2792 = Path To String(path=w3591) -> (string=w3586:string)
            "string1 3" <- w3586
            n2793 = Match Pattern(string=w3589, regular expression=".dgf") -> (before substring=→"String Control 5":string)  [unwired: 1 in, 3 out]
            n2794 = Match Pattern(string=w3586, regular expression=".dgf" ("substring (\"\")")) -> (before substring=w3596:string)  [unwired: 1 in, 3 out]
            n2795 = Concatenate Strings(w3596, ".duf" ("Substring")) -> (w3593:string)
            n2796 = String To Path(string=w3593) -> (path=w3597:path)
            n2797 = call <vilib>:"Read Characters From File.vi"("file path (dialog if empty)"=w3597, "start of read offset (chars.:0)"=60 ("start of read offset (chars.: 0)")) -> ("character string"=→"String Control 6":string)  [unwired: 4 in, 3 out]
          }
        }
        n2798 = case shown="True" "OPEN 4" {
          frame False {
          }
          frame True {
            (unwired) 0  # existing file
            w3618 = "Choose a datalog file to open"  # prompt
            n2799 = local write "OPEN 4"(FALSE ("OPEN 1")) -> ()
            n2800 = String To Path(string="C:\\LAB-IQ\\Data\\") -> (path=w3603:path)
            n2801 = File Dialog(6:"*.dgf" ("pattern"), 7:w3618, 11:w3603) -> (0:w3601:errorcluster, 3:w3609:path)  [unwired: 4 in, 2 out]
            n2802 = Unbundle(w3601) -> ()  [unwired: 3 out]
            n2803 = Strip Path(path=w3609) -> (name=w3607:string)  [unwired: 1 out]
            n2804 = Path To String(path=w3609) -> (string=w3604:string)
            "string1 4" <- w3604
            n2805 = Match Pattern(string=w3607, regular expression=".dgf") -> (before substring=→"String Control 7":string)  [unwired: 1 in, 3 out]
            n2806 = Match Pattern(string=w3604, regular expression=".dgf" ("substring (\"\")")) -> (before substring=w3614:string)  [unwired: 1 in, 3 out]
            n2807 = Concatenate Strings(w3614, ".duf" ("Substring")) -> (w3611:string)
            n2808 = String To Path(string=w3611) -> (path=w3615:path)
            n2809 = call <vilib>:"Read Characters From File.vi"("file path (dialog if empty)"=w3615, "start of read offset (chars.:0)"=60 ("start of read offset (chars.: 0)")) -> ("character string"=→"String Control 8":string)  [unwired: 4 in, 3 out]
          }
        }
      }
      frame "About" {
        # "Elapsed time\ncof\nstroke\nmean pos\nTemp\nHumidity"
        n2810 = disable-structure shown="Disabled" {
          frame Disabled {
            n2811 = case shown="True" "Export" {
              frame False {
              }
              frame True {
                w3640 = "                                      " ("string")
                w3642 = "\r"
                (unwired) i16 6 ("width (-)")
                w3719 = "\r"
                w3651 = "\r"
                n2812 = local write "Export"(FALSE ("Export")) -> ()
                n2813 = local read "String 29"() -> (w3688:string)
                n2814 = local read "String 34"() -> (w3676:string)
                n2815 = local read "String 35"() -> (w3671:string)
                n2816 = local read "String 37"() -> (w3667:string)
                n2817 = local read "String 36"() -> (w3664:string)
                n2818 = local read "String 38"() -> (w3661:string)
                n2819 = local read "String 39"() -> (w3658:string)
                n2820 = Match Pattern(string=w3688, regular expression=".dwm") -> (before substring=w3684:string)  [unwired: 1 in, 3 out]
                "before substring" <- w3684
                n2821 = local read "S 38"() -> (w3679:string)
                n2822 = local read "S 39"() -> (w3672:string)
                n2823 = local read "Temperature before test 2"() -> (w3708:dbl)
                n2824 = local read "Temperature after test 2"() -> (w3713:dbl)
                n2825 = local read "Humidity before test 2"() -> (w3694:dbl)
                n2826 = local read "Humidity after test 2"() -> (w3709:dbl)
                n2827 = local read "MWSD 2"() -> (w3705:dbl)
                n2828 = local read "WS1.4 2"() -> (w3721:dbl)
                n2829 = local read "HCF 2"() -> (w3717:dbl)
                n2830 = local read "AVP 2"() -> (w3706:dbl)
                n2831 = Concatenate Strings("1," ("string"), w3679) -> (w3678:string)
                n2832 = Concatenate Strings("2," ("string"), w3676) -> (w3675:string)
                n2833 = Concatenate Strings("3," ("string"), w3672) -> (w3674:string)
                n2834 = Concatenate Strings("4," ("string"), w3671) -> (w3670:string)
                n2835 = Concatenate Strings("5," ("string"), w3667) -> (w3668:string)
                n2836 = Concatenate Strings("6," ("string"), w3664) -> (w3665:string)
                n2837 = Concatenate Strings("7," ("string"), w3661) -> (w3662:string)
                n2838 = Concatenate Strings("8," ("string"), w3658) -> (w3659:string)
                n2839 = local read "Sample ID"() -> (w3726:string)
                n2840 = case shown="\"xlx\"" "Select File Type" {
                  tunnel: w3684 -> [w3729 w3731 w3733]
                  tunnel: [w3727 w3732 w3734] -> w3683
                  frame "xlx" {
                    n2841 = Concatenate Strings(w3729, ".xls" ("string")) -> (w3727:string)
                  }
                  frame "csv" {
                    n2842 = Concatenate Strings(w3731, ".csv" ("string")) -> (w3732:string)
                  }
                  frame "txt" {
                    n2843 = Concatenate Strings(w3733, ".txt" ("string")) -> (w3734:string)
                  }
                }
                n2844 = local read "Test Date"() -> (w3725:string)
                n2845 = local read "String 45"() -> (w3639:string)
                n2846 = local read "String 31"() -> (w3724:string)
                n2847 = local read "String 32"() -> (w3723:string)
                n2848 = local read "TITTLE"() -> (w3647:string)
                n2849 = Number To Fractional String(number=w3694, width (-)=i16 6, precision (6)=i16 2) -> (F-format string=w3693:string)  [unwired: 1 in]
                n2850 = Number To Fractional String(number=w3708, width (-)=i16 6, precision (6)=i16 2) -> (F-format string=w3714:string)  [unwired: 1 in]
                n2851 = Number To Fractional String(number=w3709, width (-)=i16 6, precision (6)=i16 2) -> (F-format string=w3707:string)  [unwired: 1 in]
                n2852 = Number To Fractional String(number=w3713, width (-)=i16 6, precision (6)=i16 2) -> (F-format string=w3712:string)  [unwired: 1 in]
                n2853 = Number To Fractional String(number=w3705, width (-)=i16 6, precision (6)=i16 2) -> (F-format string=w3703:string)  [unwired: 1 in]
                n2854 = Number To Fractional String(number=w3706, width (-)=i16 6, precision (6)=i16 2) -> (F-format string=w3704:string)  [unwired: 1 in]
                n2855 = Number To Fractional String(number=w3717, width (-)=i16 6, precision (6)=i16 2) -> (F-format string=w3718:string)  [unwired: 1 in]
                n2856 = Number To Fractional String(number=w3721, precision (6)=i16 2) -> (F-format string=w3722:string)  [unwired: 2 in]
                n2857 = local read "s.NO"() -> (w3641:string)
                n2858 = Concatenate Strings("=" ("string"), w3647) -> (w3646:string)
                n2859 = Concatenate Strings("S.No," ("string"), "                                       Parameters" ("string")) -> (w3652:string)
                n2860 = Concatenate Strings(w3719, w3678, w3693, w3719, w3675, w3714, w3719, w3674, w3707, w3719, w3670, w3712, w3719, w3668, w3703, w3719, w3665, w3704, w3719, w3662, w3718, w3719, w3659, w3722) -> (w3681:string)
                n2861 = Concatenate Strings(w3651, "," ("string"), w3639, w3641, w3640, w3723, w3726, w3640, w3724, w3725, w3651) -> (w3649:string)
                n2862 = local read "Tested by"() -> (w3655:string)
                n2863 = local read "String 33"() -> (w3656:string)
                n2864 = Concatenate Strings("," ("string"), "                                                                             " ("string")) -> (w3644:string)
                n2865 = Concatenate Strings(w3646, w3642, w3649, w3642, w3652, w3681, w3642, w3644, w3656, w3655) -> (→"export":string)
                n2866 = String To Path(string=w3683) -> (path=w3690:path)
                n2867 = local read "export"() -> (w3685:string)
                n2868 = call <vilib>:"Write Characters To File.vi"("append to file? (new file:F)"=FALSE, "character string"=w3685, "file path (dialog if empty)"=w3690) -> ()  [unwired: 2 in, 1 out]
              }
            }
          }
          frame Enabled {
          }
        }
        n2869 = case shown="True" "OK Button 17" {
          frame False {
          }
          frame True {
            (unwired) 0  # existing file
            w3943 = "Choose a datalog file to open"  # prompt
            n2870 = local write "OK Button 17"(FALSE ("OK Button 17")) -> ()
            n2871 = local read "String"() -> (w3938:string)
            n2872 = String To Path(string=w3938) -> (path=w3939:path)
            n2873 = File Dialog(6:"*.duf" ("pattern"), 7:w3943, 11:w3939) -> (0:w3930:errorcluster, 3:w3949:path)  [unwired: 4 in, 2 out]
            n2874 = Unbundle(w3930) -> ()  [unwired: 3 out]
            n2875 = Open/Create/Replace File "Open File"(file path (use dialog)=w3949) -> (refnum out=w3941:refnum<file>)  [unwired: 5 in, 2 out]
            n2876 = Strip Path(path=w3949) -> (name=w3947:string)  [unwired: 1 out]
            n2877 = Path To String(path=w3949) -> (string=w3932:string)
            n2878 = while {
              tunnel: w3941 -> [w3953]
              i -> [w3950]
              stop <- w3951 continue-if-true
              (unwired) TRUE ("line mode (F)")
              n2879 = Read from Text File "Read File"(file (use dialog)=w3953) -> (text=w3952:string)  [unwired: 3 in, 3 out]
              n2880 = local write "Numeric 16"(w3950) -> ()
              n2881 = String Length(string=w3952) -> (length=w3955:i32)
              n2882 = Greater?(x=w3955, y=1) -> (0:w3951:bool)
            }
            n2883 = local write "String 29"(w3932) -> ()
            n2884 = Search and Replace String(input string=w3932, search string=".duf", replace string=".dgf" ("replace string (\"\")")) -> (result string=→"String Indicator 4":string)  [unwired: 5 in, 3 out]
            n2885 = Match Pattern(string=w3947, regular expression=".dwm") -> (before substring=w3931:string)  [unwired: 1 in, 3 out]
            "String Indicator" <- w3931
            n2886 = Match Pattern(string=w3932, regular expression=".dwm" ("substring (\"\")")) -> (before substring=w3933:string)  [unwired: 1 in, 3 out]
            "String Indicator 3" <- w3933
            n2887 = local write "TITTLE 2"(w3931) -> ()
            n2888 = String To Path(string=w3933) -> (path=w3940:path)
            "path" <- w3940
            n2889 = call <vilib>:"Read Characters From File.vi"("file path (dialog if empty)"=w3940, "start of read offset (chars.:0)"=60 ("start of read offset (chars.: 0)")) -> ("character string"=→"String Indicator 2":string)  [unwired: 4 in, 3 out]
          }
        }
        n2890 = call <vilib>:"Query Available Printers.vi"() -> ("system configured printers"=w3632:string[])  [unwired: 9 in, 2 out]
        "System Configured Printers 2" <- w3632
        n2891 = local read "OK Button 16"() -> (w3629:bool)
